vi "CAN Filter Messages.vi"(7 "Mode":u8, 9 "ToID":u32, 10 "FromID":u32, 11 "Channel":u16) -> (3 "function return":u32)   [LabVIEW 2020, in "PCANBasic.lvlib"]
doc: "TPCANStatus __stdcall CAN_FilterMessages(\n TPCANHandle Channel, \n DWORD FromID, \n DWORD ToID, \n TPCANMode Mode);"
uses:
  PCANBasic.lvlib
  <userlib>/PCANBasic/PCANBasic.dll
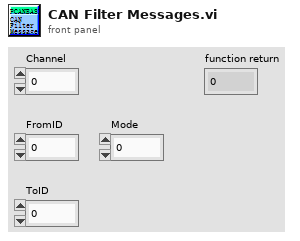
[diagram p1: front panel]
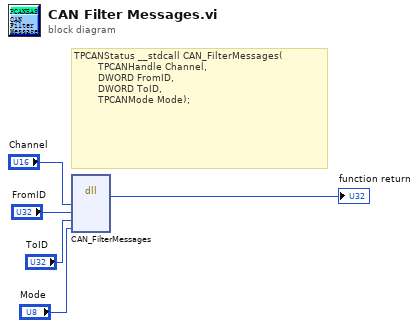
[diagram p0: block diagram]
diagram:
  # "TPCANStatus __stdcall CAN_FilterMessages(\n        TPCANHandle Channel, \n        DWORD FromID, \n        DWORD ToID, \n        TPCANMode Mode);"
  n1 = dll-call lib="D:/Program Files (x86)/National Instruments/LabVIEW 2020/user.lib/PCANBasic/PCANBasic.*" fn="CAN_FilterMessages"("Channel"="Channel", "FromID"="FromID", "ToID"="ToID", "Mode"="Mode") -> (→"function return":u32)  [unwired: 7 in, 2 out]
